vi "GetLastGuess.vi"(8 "error in (no error)":errorcluster, 11 "View in":refnum<class "View.lvclass">) -> (0 "error out":errorcluster, 1 "Letters":string[](array[string]), 2 "Last Guess":string, 3 "View out":refnum<class "View.lvclass">)   [LabVIEW 2024, in "GUI.lvlib" / "View.lvclass"]
uses:
  View.lvclass
  View.lvclass/View.ctl
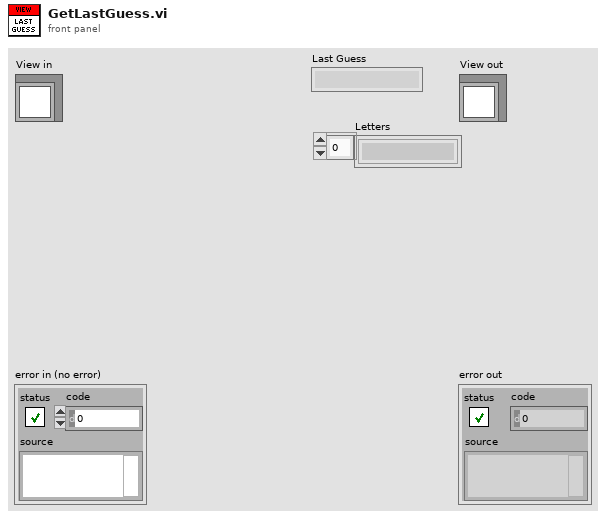
[diagram p1: front panel]
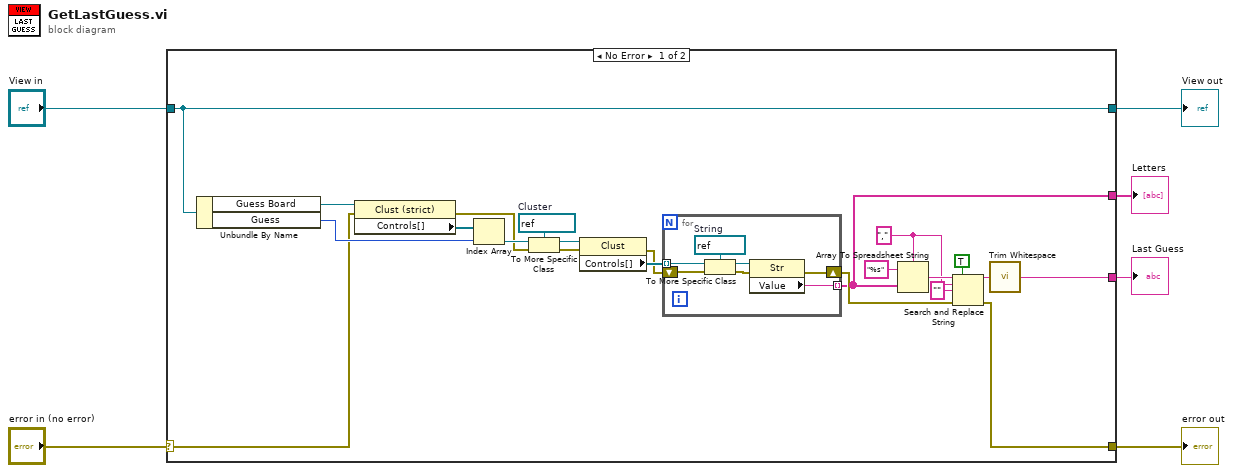
[diagram p0: block diagram]
diagram:
  n1 = case shown="No Error" "error in (no error)" {
    selector: "error in (no error)" -> [w14 w37]
    tunnel: [w9 w37] -> w5
    tunnel: [w15 w36] -> w3
    tunnel: "View in" -> [w15 w36]
    tunnel: [w8 _] -> w2
    tunnel: [w7 _] -> w1
    frame No Error {
      w20 = "," ("delimiter (Tab)")
      w25 = refnum<vi> refnum  # Cluster
      n2 = Unbundle By Name(w15) -> ("Guess Board"=w28:refnum<vi>, "Guess"=w16:i32)
      n3 = property class="Clust (strict)"(reference=w28, error in=w14) -> (error out=w13:errorcluster, "Controls[]"=w27:refnum<vi>[])  [unwired: 1 out]
      n4 = Index Array(array=w27, index=w16) -> (element=w26:refnum<vi>)
      n5 = To More Specific Class(target class=w25, reference=w26, error in=w13) -> (specific class reference=w24:refnum<vi>, error out=w12:errorcluster)
      n6 = property class="Clust"(reference=w24, error in=w12) -> (error out=w11:errorcluster, "Controls[]"=w23:refnum<vi>[])  [unwired: 1 out]
      n7 = for {
        tunnel: w23 -> [w35] mode=indexing
        shift-right: [w30] -> w10
        shift-left: w11 -> [w33]
        tunnel: [w29] -> w7 mode=indexing
        w34 = refnum<vi> refnum  # String
        n8 = To More Specific Class(target class=w34, reference=w35, error in=w33) -> (specific class reference=w31:refnum<vi>, error out=w32:errorcluster)
        n9 = property class="Str"(reference=w31, error in=w32) -> (error out=w30:errorcluster, "Value"=w29:string)  [unwired: 1 out]
      }
      n10 = Array To Spreadsheet String(delimiter (Tab)=w20, array=w7, 3:"%s" ("format string")) -> (spreadsheet string=w21:string)
      n11 = Search and Replace String(replace all?=TRUE ("replace all? (F)"), input string=w21, search string=w20, replace string="" ("replace string (\"\")"), error in=w10) -> (result string=w17:string, error out=w9:errorcluster)  [unwired: 3 in, 2 out]
      n12 = call <vilib>:"Trim Whitespace.vi"("string"=w17) -> ("trimmed string"=w8:string)  [unwired: 1 in]
    }
    frame Error {
    }
  }
  "error out" <- w5
  "View out" <- w3
  "Last Guess" <- w2
  "Letters" <- w1
